vi "Configure Common.vi"(0 "Instrument Handle In":refnum<k21>, 1 "Selector String":string, 5 "Common Configuration":T1={"Measurement Interval (s)"=0.0001, "Signal Type"=0, "DUT Average Input Power (dBm)"=-15.0, "Synchronization Method"=1} {"Synchronization Method" items=["Direct"=1, "Alias Protected"=2]; "DUT Average Input Power (dBm)" format="%.2f"; "Signal Type" items=["Modulated", "Tones"]; "Measurement Interval (s)" format="%#.2p"}, 7 "Reference Waveform":T2={"Name"="Wfm", "Data"=refnum, "Signal Bandwidth (Hz)"=0.0, "PAPR (dB)"=0.0, "Burst Length (s)"=0.0, "Sample Rate"=0.0, "Burst Start Locations"=[], "Burst Stop Locations"=[], "Idle Duration Present?"=FALSE, "Runtime Scaling"=0.0, "Script"=""} {"Runtime Scaling" format="%#_6p"; "Sample Rate" format="%#_6p"; "Burst Length (s)" format="%#_6p"; "PAPR (dB)" format="%.2f"; "Signal Bandwidth (Hz)" format="%#_6p"}, 11 "error in (no error)":errorcluster) -> (4 "Instrument Handle Out":refnum<k21>, 15 "error out":errorcluster)   [LabVIEW 2019, in "RFmxDPD.lvlib"]
doc: "Configures common settings for the application of DPD, regardless of which model is used."
uses:
  RFmxDPD.lvlib
  Common/Waveform.ctl
  Typedefs/Common Configuration.ctl
  <vilib>/RFmx/SpecAn/mx/RFmxSpecAn.llb/RFmxSpecAn Select Measurement (Single).vi
  Common/Common.lvlib
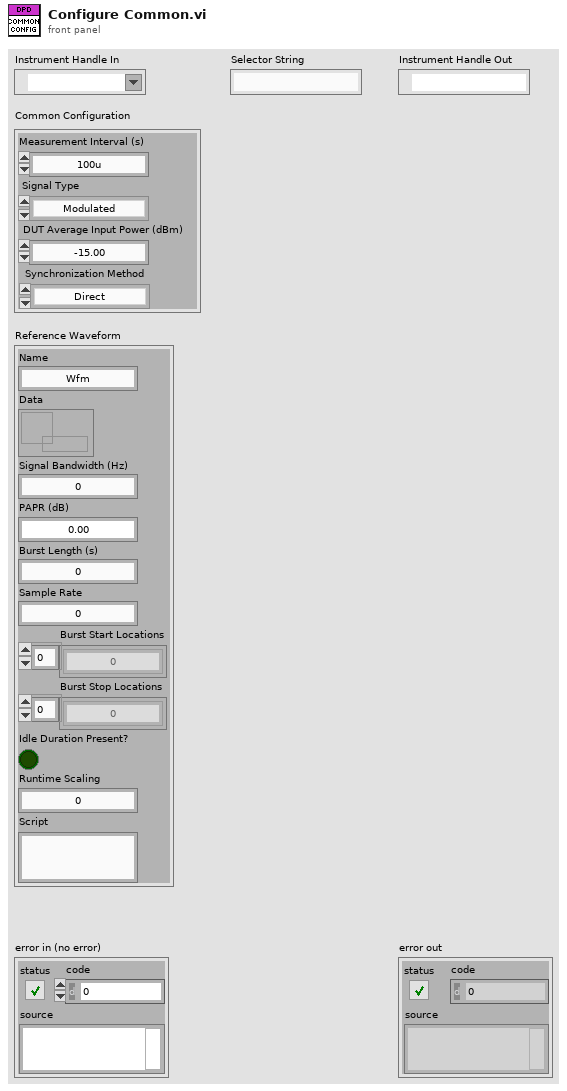
[diagram p1: front panel]
types:
  T1 = typedef "RFmxDPD.lvlib/Common Configuration.ctl" = cluster{"Measurement Interval (s)":dbl, "Signal Type":i32, "DUT Average Input Power (dBm)":dbl, "Synchronization Method":i32}
  T2 = typedef "Common.lvlib/Waveform.ctl" = cluster{"Name":string, "Data":refnum<data-value>, "Signal Bandwidth (Hz)":dbl, "PAPR (dB)":dbl, "Burst Length (s)":dbl, "Sample Rate":dbl, "Burst Start Locations":i32[], "Burst Stop Locations":i32[], "Idle Duration Present?":bool, "Runtime Scaling":dbl, "Script":string}
  T3 = enum16{"ACP", "CCDF", "CHP", "FCnt", "Harmonics", "OBW", "SEM", "Spectrum", "Spur", "TXP", "AMPM", "DPD", "IQ", "IM", "NF", "PhaseNoise", "PAVT"}
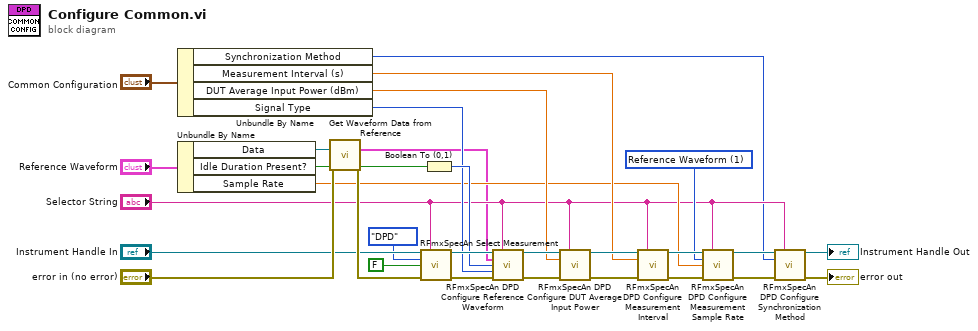
[diagram p0: block diagram]
diagram:
  w9 = 1 items=["User", "Reference Waveform"] ("Sample Rate Mode")
  n1 = Unbundle By Name("Common Configuration") -> ("Synchronization Method"=w5:i32, "Measurement Interval (s)"=w11:dbl, "DUT Average Input Power (dBm)"=w12:dbl, "Signal Type"=w13:i32)
  n2 = Unbundle By Name("Reference Waveform") -> ("Data"=w16:refnum<data-value>, "Idle Duration Present?"=w15:bool, "Sample Rate"=w8:dbl)
  n3 = call "Get Waveform Data from Reference.vi"("Waveform Data Reference"=w16, "error in (no error)"="error in (no error)") -> ("Waveform Data"=w2:cluster{"t0":dbl, "dt":dbl, "y":csg[]}, "error out"=w23:errorcluster)  [unwired: 12 in]
  n4 = call-poly <vilib>:"RFmxSpecAn Select Measurement.vi"("Instrument Handle In"="Instrument Handle In", "Selector String"="Selector String", "Measurement"=T3."DPD", "Enable All Traces"=FALSE, "error in (no error)"=w23) -> ("Instrument Handle Out"=w21:refnum<k21>, "error out"=w30:errorcluster)  [unwired: 9 in]
  n5 = Boolean To (0,1)(Boolean=w15) -> (0, 1=w14:i16)
  n6 = call <vilib>:"RFmxSpecAn DPD Configure Reference Waveform.vi"("Instrument Handle In"=w21, "Selector String"="Selector String", "Reference Waveform"=w2, "Idle Duration Present"=w14, "Signal Type"=w13, "error in (no error)"=w30) -> ("Instrument Handle Out"=w20:refnum<k21>, "error out"=w29:errorcluster)  [unwired: 8 in]
  n7 = call <vilib>:"RFmxSpecAn DPD Configure DUT Average Input Power.vi"("Instrument Handle In"=w20, "Selector String"="Selector String", "DUT Average Input Power (dBm)"=w12, "error in (no error)"=w29) -> ("Instrument Handle Out"=w19:refnum<k21>, "error out"=w28:errorcluster)  [unwired: 10 in]
  n8 = call <vilib>:"RFmxSpecAn DPD Configure Measurement Interval.vi"("Instrument Handle In"=w19, "Selector String"="Selector String", "Measurement Interval (s)"=w11, "error in (no error)"=w28) -> ("Instrument Handle Out"=w18:refnum<k21>, "error out"=w27:errorcluster)  [unwired: 10 in]
  n9 = call <vilib>:"RFmxSpecAn DPD Configure Measurement Sample Rate.vi"("Instrument Handle In"=w18, "Selector String"="Selector String", "Sample Rate Mode"=w9, "Sample Rate (S/s)"=w8, "error in (no error)"=w27) -> ("Instrument Handle Out"=w7:refnum<k21>, "error out"=w25:errorcluster)  [unwired: 9 in]
  n10 = call <vilib>:"RFmxSpecAn DPD Configure Synchronization Method.vi"("Instrument Handle In"=w7, "Selector String"="Selector String", "Synchronization Method"=w5, "error in (no error)"=w25) -> ("Instrument Handle Out"=→"Instrument Handle Out":refnum<k21>, "error out"=→"error out":errorcluster)  [unwired: 10 in]
